vi "Get Address Map Element.vi"(2 "AO in":refnum<class "AO1.lvclass">, 5 "index":u8) -> (6 "address map element":T1)   [LabVIEW 2017, in "Analog IO.lvlib" / "AO1.lvclass"]
uses:
  AO1.lvclass
  <instrlib>/_niInstr/Instruction Framework/v1/FPGA/Typedefs/Address Map Element.ctl
  <instrlib>/_niInstr/Instruction Framework/v1/FPGA/Typedefs/niInstr Instruction Framework v1 FPGA.lvlib
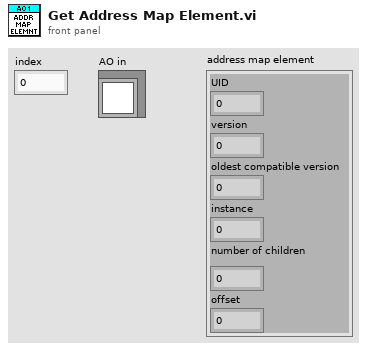
[diagram p1: front panel]
types:
  T1 = typedef "niInstr Instruction Framework v1 FPGA.lvlib/Address Map Element.ctl" = cluster{"UID":u16, "version":u16, "oldest compatible version":u16, "instance":u8, "number of children":u8, "offset":u32}
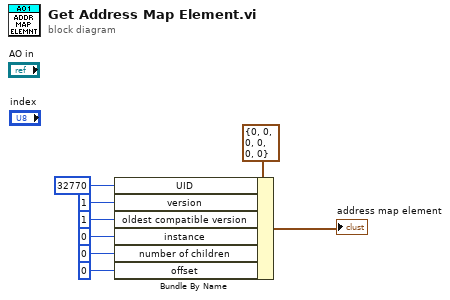
[diagram p0: block diagram]
diagram:
  n1 = Bundle By Name(cluster=T1 {"UID"=0, "version"=0, "oldest compatible version"=0, "instance"=0, "number of children"=0, "offset"=0} ("address map element"), "UID"=u16 32770, "version"=u16 1, "oldest compatible version"=u16 1, "instance"=u8 0, "number of children"=u8 0, "offset"=u32 0) -> (→"address map element":T1)
